vi "Ex-02 Acq Finite Multipoint.vi"() -> ()   [LabVIEW 2012]
doc: "© Copyright M. Ferrari 2012 \nMultipoint Analog Acq. Template"
uses:
  <vilib>/DAQmx/configure/timing.llb/DAQmx Timing (Sample Clock).vi
  <vilib>/DAQmx/create/channels.llb/DAQmx Create Channel (AI-Voltage-Basic).vi
  <vilib>/DAQmx/read.llb/DAQmx Read (Analog Wfm 1Chan NSamp).vi
panel:
  out "Volt Graph":waveform(dbl)(graph)
  in  "n° samples":i32=100
  in  "rate":dbl=10000.0
  in  "min":dbl=-5.0 format="%0.2f"
  in  "max":dbl=5.0 format="%0.2f"
  in  "in conf":i32(ring)=10083 items=["default"=-1, "RSE"=10083, "NRSE"=10078, "Differential"=10106, "Pseudodifferential"=12529]
  in  "physical ch":tag="Dev1/ai0"
  # "RANGE"
  # "rate specifies the sampling rate in samples per channel per second. \nIf you use an external source for the Sample Clock, \nset this input to the maximum expected rate of that clock."
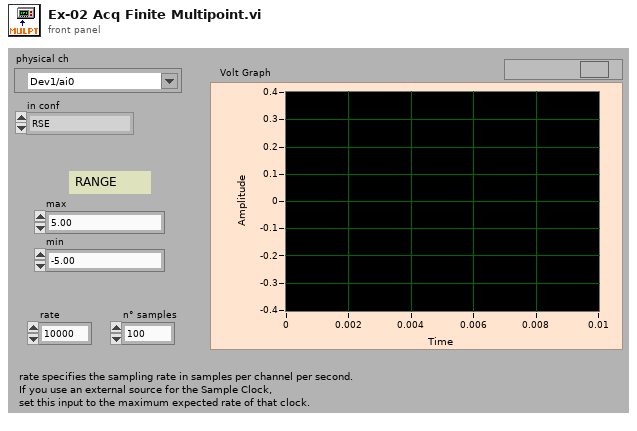
[diagram p1: front panel]
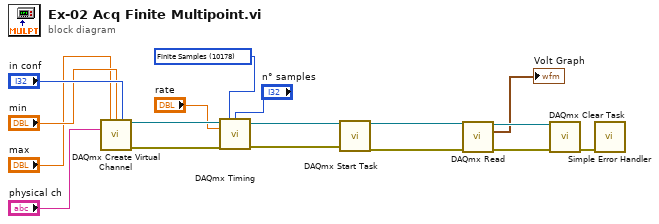
[diagram p0: block diagram]
diagram:
  w6 = 10178 items=["Finite Samples"=10178, "Continuous Samples"=10123, "Hardware Timed Single Point"=12522] ("sample mode")
  n1 = call-poly <vilib>:"DAQmx Create Virtual Channel.vi"("maximum value"="max", "minimum value"="min", "input terminal configuration"="in conf", "physical channels"="physical ch") -> ("task out"=w12:refnum<k21>, "error out"=w10:errorcluster)  [unwired: 10 in]
  n2 = call-poly <vilib>:"DAQmx Timing.vi"("task/channels in"=w12, "sample mode"=w6, "samples per channel"="n° samples", "rate"="rate", "error in"=w10) -> ("task out"=w11:refnum<k21>, "error out"=w9:errorcluster)  [unwired: 2 in, 7 out]
  n3 = call <vilib>:"DAQmx Start Task.vi"("task/channels in"=w11, "error in"=w9) -> ("task out"=w2:refnum<k21>, "error out"=w3:errorcluster)  [unwired: 12 out]
  n4 = call-poly <vilib>:"DAQmx Read.vi"("task/channels in"=w2, "error in"=w3) -> ("task out"=w5:refnum<k21>, "data"=→"Volt Graph":waveform(dbl), "error out"=w4:errorcluster)  [unwired: 1 in, 10 out]
  n5 = call <vilib>:"DAQmx Clear Task.vi"("task in"=w5, "error in"=w4) -> ("error out"=w17:errorcluster)  [unwired: 13 out]
  n6 = call <vilib>:"Simple Error Handler.vi"("error in (no error)"=w17) -> ()  [unwired: 1 in, 8 out]
